vi "CMD and expected feedback.vi"(9 "f in":i32, 10 "y":string, 11 "string":string) -> (3 "f out":i32)   [LabVIEW 2012]
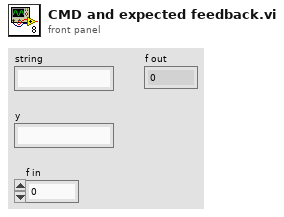
[diagram p1: front panel]
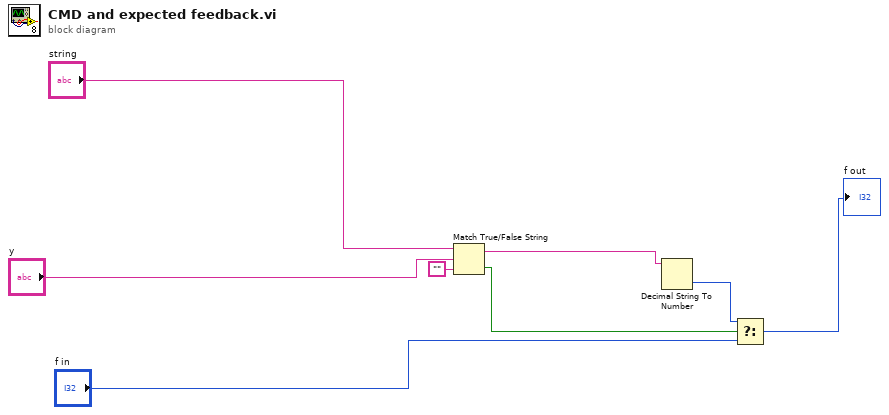
[diagram p0: block diagram]
diagram:
  n1 = Match True/False String(2:"" ("false string"), 3:"y", 4:"string") -> (0:w5:bool, 1:w1:string)
  n2 = Decimal String To Number(string=w1) -> (number=w6:i32)  [unwired: 2 in, 1 out]
  n3 = Select(t=w6, s=w5, f="f in") -> (s? t:f=→"f out":i32)
